vi "Exit.vi"(8 "error in (no error)":errorcluster, 11 "VI Refnum":refnum<vi>) -> (0 "error out":errorcluster)   [LabVIEW 2019]
uses:
  Message Queue/Message Queue.lvlib
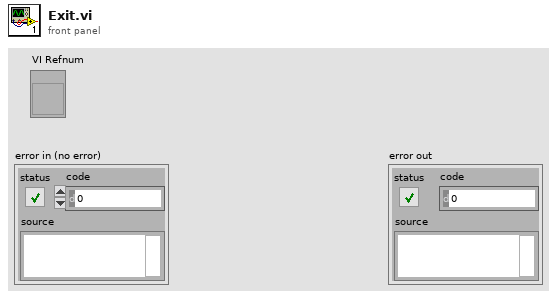
[diagram p1: front panel]
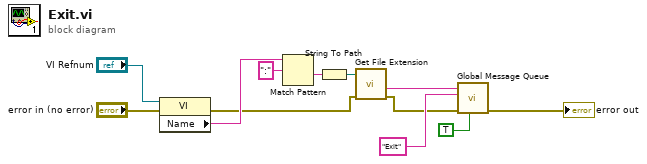
[diagram p0: block diagram]
diagram:
  n1 = property class="VI"(reference="VI Refnum", error in="error in (no error)") -> (error out=w2:errorcluster, "Name"=w4:string)  [unwired: 1 out]
  n2 = Match Pattern(string=w4, regular expression=":") -> (after substring=w6:string)  [unwired: 1 in, 3 out]
  n3 = String To Path(string=w6) -> (path=w5:path)
  n4 = call <vilib>:"Get File Extension.vi"("error in (no error)"=w2, "file"=w5) -> ("error out"=w1:errorcluster, "filename without extension"=w3:string)  [unwired: 5 in, 3 out]
  n5 = call "Global Message Queue.vi"("Priority?"=TRUE, "error in (no error)"=w1, "State Name"="Exit", "Module Name"=w3) -> ("error out"=→"error out":errorcluster)  [unwired: 7 in]
